vi "Vision Processing.vi"(7 "CameraDevRef":T1) -> ()   [LabVIEW 2011]
doc: "This VI runs in parallel to other tasks. It gets images from the camera, processes them for color or shape and use that information to affect robot behavior."
uses:
  <vilib>/Rock Robotics/WPI/Camera/WPI_CameraDevRef.ctl
  Robot Global Data.vi
  <vilib>/vision/NI_Vision_Development_Module.lvlib
panel:
  out "Distance Array":dbl[](array[numeric])
  out "Distance to Midpoint":dbl
  in  "Scaler":dbl=0.5
  in  "Enable Imaging on Screen":bool
  out "Midpoint":dbl
  in  "Lower Speed Limit":dbl=0.05
  out "Turret Rotation":dbl
  in  "Upper Speed Limit":dbl=0.3
  out "Number of Rectangles Visible":dbl
  out "Y Position Array":dbl[](array[numeric])
  out "X Position Array":dbl[](array[numeric])
  out "Array":T2(array[cluster])
  in  "Score Limits":T3={"Rect Coverage"=76.0, "Aspect Ratio"=40.0, "X Edge Strength"=40.0, "Y Edge Strength"=60.0}
  out "Processed Image":T4(plugin-control)
  out "Original Image":T4(plugin-control)
  in  "Annotate":bool=TRUE
  in  "Particle Count Limit":i32=10
  in  "Area Size Limit":i32=444
  in  "Range":cluster{"Lower value":sgl, "Upper value":sgl}={"Lower value"=120.0, "Upper value"=255.0}
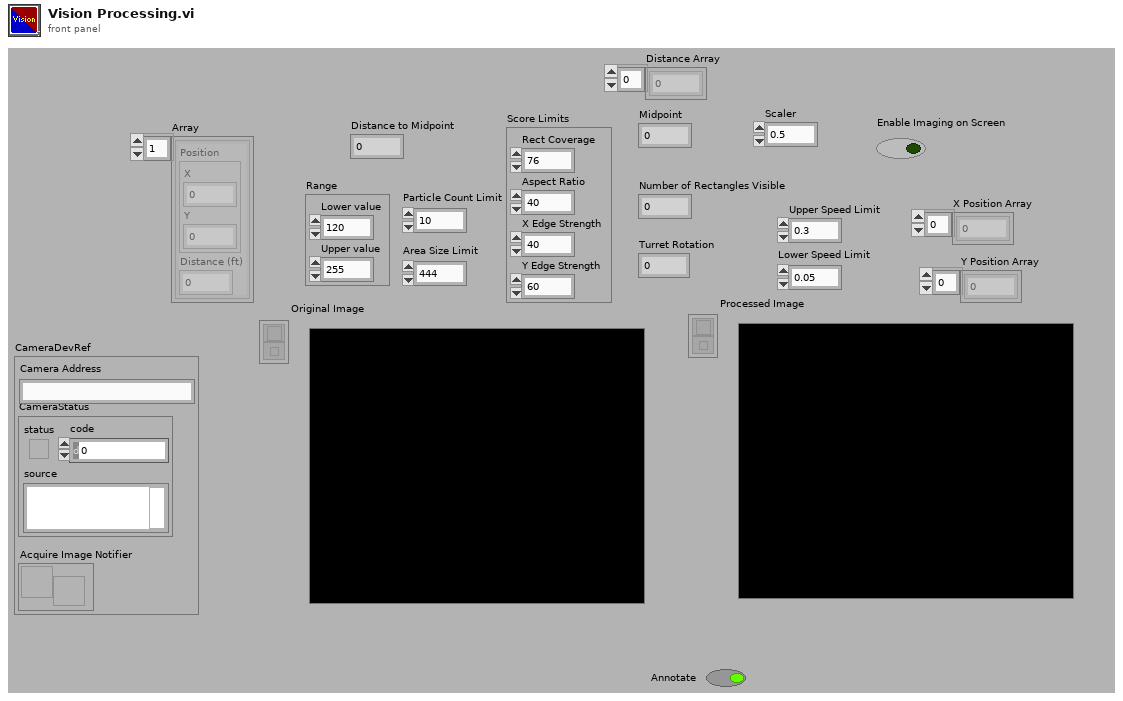
[diagram p1: front panel]
types:
  T1 = typedef "WPI_CameraDevRef.ctl" = cluster{"Camera Address":string, "CameraStatus":errorcluster, "Acquire Image Notifier":refnum<notifier>}
  T2 = cluster{"Position":cluster{"X":dbl, "Y":dbl}, "Distance (ft)":dbl}[]
  T3 = cluster{"Rect Coverage":dbl, "Aspect Ratio":dbl, "X Edge Strength":dbl, "Y Edge Strength":dbl}
  T4 = typedef "IMAQ Image.ctl" = refnum<image>
  T5 = typedef "Image Type" = u32
  T6 = cluster{cluster{"Left":dbl, "Top":dbl, "Right":dbl, "Bottom":dbl}, dbl[]}[]
  T7 = cluster{"Left":dbl, "Top":dbl, "Right":dbl, "Bottom":dbl}
  T8 = cluster{"Target Center (-1 to 1)":cluster{"X":dbl, "Y":dbl}, "Distance (ft)":dbl}
  T9 = cluster{"Target Center (-1 to 1)":cluster{"X":dbl, "Y":dbl}, "Distance (ft)":dbl}[]
  T10 = cluster{"Axis 1":dbl, "Axis 2":dbl, "Axis 3":dbl, "Axis 4":dbl, "Axis 5":dbl, "Axis 6":dbl, "Button 1":bool, "Button 2":bool, "Button 3":bool, "Button 4":bool, "Button 5":bool, "Button 6":bool, "Button 7":bool, "Button 8":bool, "Button 9":bool, "Button 10":bool, "Button 11":bool, "Button 12":bool}
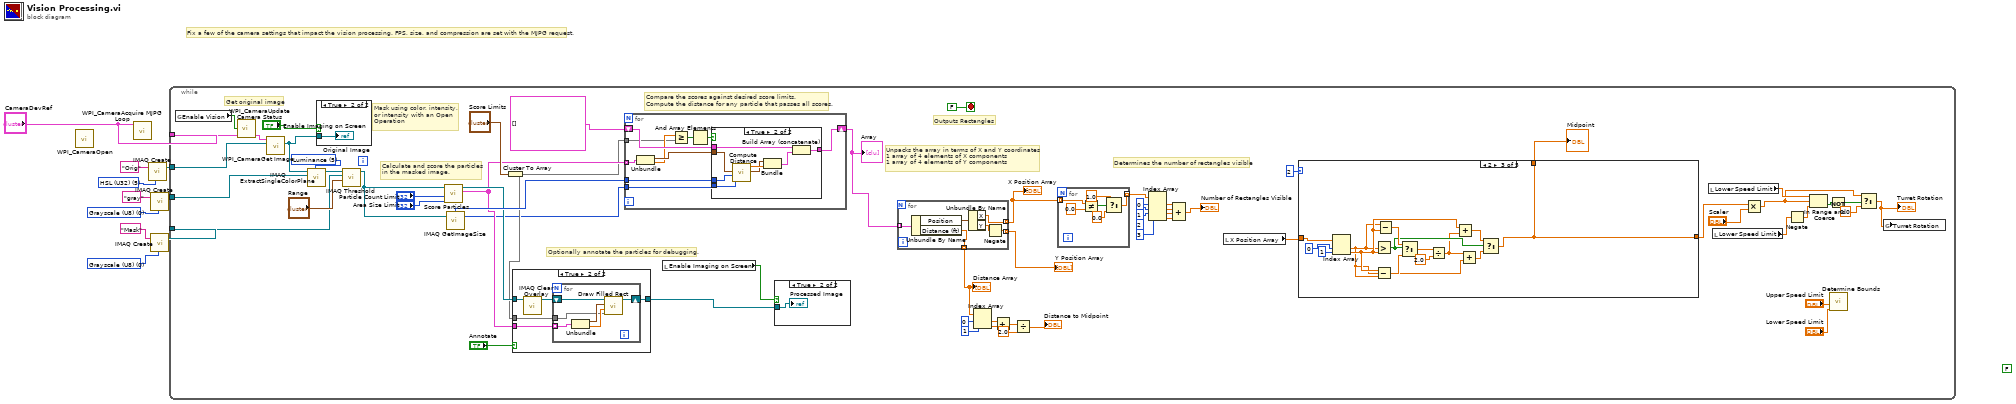
[diagram p0: block diagram]
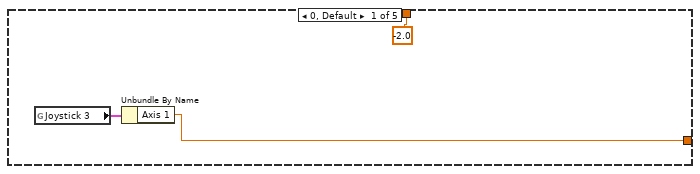
[diagram p4: hidden frame]
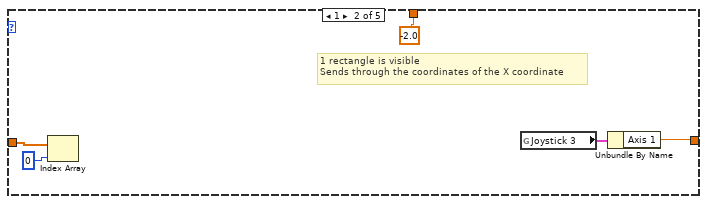
[diagram p5: hidden frame]
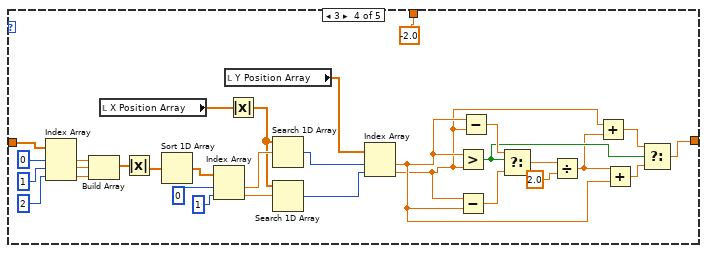
[diagram p6: hidden frame]
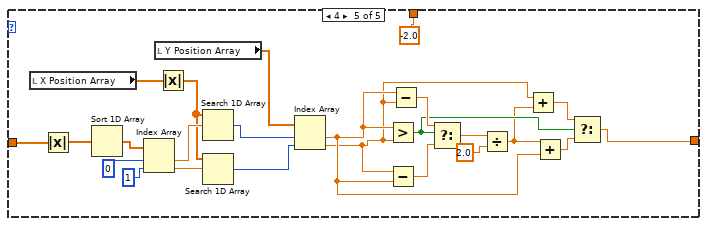
[diagram p7: hidden frame]
diagram:
  w3 = T5 5 items=["Grayscale (U8)", "Grayscale (I16)", "Grayscale (SGL)", "Complex (CSG)", "RGB (U32)", "HSL (U32)", "RGB (U64)", "Grayscale (U16)"] ("Image Type")
  (unwired) FALSE
  w6 = T5 0 items=["Grayscale (U8)", "Grayscale (I16)", "Grayscale (SGL)", "Complex (CSG)", "RGB (U32)", "HSL (U32)", "RGB (U64)", "Grayscale (U16)"] ("Image Type")
  w10 = T5 0 items=["Grayscale (U8)", "Grayscale (I16)", "Grayscale (SGL)", "Complex (CSG)", "RGB (U32)", "HSL (U32)", "RGB (U64)", "Grayscale (U16)"] ("Image Type")
  # "Fix a few of the camera settings that impact the vision processing. FPS, size, and compression are set with the MJPG request."
  n1 = call <vilib>:"WPI_CameraOpen.vi"() -> ()  [unwired: 10 in, 2 out]
  n2 = call <vilib>:"WPI_CameraAcquire MJPG Loop.vi"("CameraDevRef"="CameraDevRef") -> ()  [unwired: 11 in]
  n3 = call "IMAQ Create"("Image Name"="Orig", "Image Type"=w3) -> ("New Image"=w2:T4)  [unwired: 2 in, 2 out]
  n4 = call "IMAQ Create"("Image Name"="gray", "Image Type"=w10) -> ("New Image"=w8:T4)  [unwired: 2 in, 2 out]
  n5 = call "IMAQ Create"("Image Name"="Mask", "Image Type"=w6) -> ("New Image"=w5:T4)  [unwired: 2 in, 2 out]
  n6 = while {
    tunnel: w8 -> [w56]
    tunnel: w5 -> [w57]
    tunnel: w2 -> [w35]
    tunnel: "CameraDevRef" -> [w33]
    stop <- FALSE stop-if-true
    w60 = 5 items=["Red", "Green", "Blue", "Hue", "Saturation", "Luminance", "Value", "Intensity"] ("Color Plane")
    # "Determines the number of rectangles visible"
    # "Unpacks the array in terms of X and Y coordinates\n1 array of 4 elements of X components\n1 array of 4 elements of Y components"
    # "Outputs Rectangles"
    # "Optionally annotate the particles for debugging."
    # "Compare the scores against desired score limits.\nCompute the distance for any particle that passes all scores."
    # "Calculate and score the particles\nin the masked image."
    # "Mask using color, intensity,\nor intensity with an Open\nOperation"
    # "Get original image"
    n7 = global read "Robot Global Data.vi" "Enable Vision"() -> (w32:bool)
    n8 = call <vilib>:"WPI_CameraUpdate Camera Status.vi"("CameraDevRef In"=w33, "Enable Vision"=w32) -> ("CameraDevRef Out"=w34:T1)  [unwired: 3 in]
    n9 = call <vilib>:"WPI_CameraGet Image.vi"("Image"=w35, "CameraDevRef"=w34) -> ("Image Out"=w31:T4)  [unwired: 7 in, 2 out]
    n10 = call "IMAQ ExtractSingleColorPlane"("Color Plane"=w60, "Image Dst"=w56, "Image Src"=w31) -> ("Image Dst Out"=w58:T4)  [unwired: 1 in, 7 out]
    n11 = case shown="True" "Enable Imaging on Screen" {
      tunnel: w31 -> [_ w73]
      frame False {
      }
      frame True {
        "Original Image" <- w73
      }
    }
    n12 = call "IMAQ Threshold"("Range"="Range", "Image Dst"=w57, "Image Src"=w58) -> ("Image Dst Out"=w55:T4)  [unwired: 3 in, 5 out]
    n13 = call "Score Particles.vi"("Area Size Limit"="Area Size Limit", "Particle Count Limit"="Particle Count Limit", "Image Refnum in"=w55) -> ("Scored Particle Info"=w67:T6, "Image Refnum out"=w70:T4)  [unwired: 7 in]
    n14 = call "IMAQ GetImageSize"("Image"=w55) -> ("Y Resolution"=w61:i32, "X Resolution"=w71:i32)  [unwired: 3 in, 1 out]
    n15 = Cluster To Array(cluster="Score Limits") -> (array=w65:dbl[])
    n16 = case shown="True" "Annotate" {
      tunnel: w70 -> [w163 w168]
      tunnel: [w163 w167] -> w68
      tunnel: w67 -> [_ w165]
      tunnel: w65 -> [_ w164]
      frame False {
      }
      frame True {
        n17 = call "IMAQ Clear Overlay"("Image"=w168) -> ("Image Out"=w166:T4)  [unwired: 2 in, 8 out]
        n18 = for {
          shift-right: [w173] -> w167
          shift-left: w166 -> [w174]
          tunnel: w165 -> [w170] mode=indexing
          tunnel: w164 -> [w169]
          n19 = Unbundle(w170) -> (w171:T7, w172:dbl[])
          n20 = call "Draw Filled Rect.vi"("Limits"=w169, "Scores"=w172, "Bounding Box"=w171, "image in"=w174) -> ("image out"=w173:T4)  [unwired: 7 in]
        }
      }
    }
    n21 = for {
      shift-right: [w183] -> w36
      shift-left: T2 [] -> [w184]
      tunnel: w71 -> [w182]
      tunnel: w67 -> [w180] mode=indexing
      tunnel: w65 -> [w176]
      tunnel: w61 -> [w175]
      n22 = Unbundle(w180) -> (w181:T7, w177:dbl[])
      n23 = Greater Or Equal?(x=w177, y=w176) -> (x >= y?=w179:bool[])
      n24 = And Array Elements(Boolean array=w179) -> (logical AND=w178:bool)
      n25 = case shown="True" w178 {
        tunnel: w184 -> [w185 w193]
        tunnel: [w185 w192] -> w183
        tunnel: w181 -> [_ w188]
        tunnel: w182 -> [_ w190]
        tunnel: w175 -> [_ w186]
        frame False {
        }
        frame True {
          n26 = call "Compute Distance.vi"("Y Image Resolution"=w186, "X Image Resolution"=w190, "Bounding Box"=w188) -> ("Target Center (-1 to 1)"=w187:cluster{"X":dbl, "Y":dbl}, "Distance (ft)"=w189:dbl)  [unwired: 7 in]
          n27 = Bundle("Target Center (-1 to 1)"=w187, "Distance (ft)"=w189) -> (w191:T8)  [unwired: 1 in]
          n28 = Build Array (concatenate)(w193, w191) -> (w192:T9)
        }
      }
    }
    "Array" <- w36
    n29 = local read "Enable Imaging on Screen"() -> (w29:bool)
    n30 = case shown="True" w29 {
      tunnel: w68 -> [_ w72]
      frame False {
      }
      frame True {
        "Processed Image" <- w72
      }
    }
    n31 = for {
      tunnel: [w160] -> w49 mode=indexing
      tunnel: [w161] -> w38 mode=indexing
      tunnel: w36 -> [w158] mode=indexing
      tunnel: [w157] -> w18 mode=indexing
      n32 = Unbundle By Name(w158) -> ("Position"=w162:cluster{"X":dbl, "Y":dbl}, "Distance (ft)"=w157:dbl)
      n33 = Unbundle By Name(w162) -> ("X"=w161:dbl, "Y"=w159:dbl)
      n34 = Negate(x=w159) -> (-x=w160:dbl)
    }
    "X Position Array" <- w38
    "Y Position Array" <- w49
    "Distance Array" <- w18
    n35 = Index Array(array=w18, index #1=0 ("index"), index #2=1 ("index")) -> (element #1=w14:dbl, element #2=w15:dbl)
    n36 = Add(x=w14, y=w15) -> (x+y=w13:dbl)
    n37 = Divide(x=w13, y=2.0) -> (x/y=→"Distance to Midpoint":dbl)
    n38 = for {
      tunnel: w38 -> [w78] mode=indexing
      tunnel: [w74] -> w39 mode=indexing
      n39 = Not Equal?(x=w78, y=0.0) -> (x != y?=w77:bool)
      n40 = Select(t=1.0, s=w77, f=0.0) -> (s? t:f=w74:dbl)
    }
    n41 = Index Array(array=w39, index #1=0 ("index"), index #2=1 ("index"), index #3=2 ("index"), index #4=3 ("index")) -> (element #1=w41:dbl, element #2=w40:dbl, element #3=w42:dbl, element #4=w43:dbl)
    n42 = Compound Arithmetic op=ADD(w41, w40, w42, w43) -> (→"Number of Rectangles Visible":dbl)
    n43 = local read "X Position Array"() -> (w37:dbl[])
    n44 = case shown="2" 2 {
      tunnel: w37 -> [_ w87 w101 w132 w136]
      tunnel: [w81 w84 w88 w104 w135] -> w22
      tunnel: [-2.0 -2.0 w88 -2.0 -2.0] -> w52
      frame 0, Default {
        n45 = global read "Robot Global Data.vi" "Joystick 3"() -> (w82:T10)
        n46 = Unbundle By Name(w82) -> ("Axis 1"=w81:dbl)
      }
      frame 1 {
        # "1 rectangle is visible\nSends through the coordinates of the X coordinate"
        n47 = Index Array(array=w87, index=0) -> ()  [unwired: 1 out]
        n48 = global read "Robot Global Data.vi" "Joystick 3"() -> (w85:T10)
        n49 = Unbundle By Name(w85) -> ("Axis 1"=w84:dbl)
      }
      frame 2 {
        n50 = Index Array(array=w101, index #1=0 ("index"), index #2=1 ("index")) -> (element #1=w89:dbl, element #2=w90:dbl)
        n51 = Greater?(x=w89, y=w90) -> (0:w94:bool)
        n52 = Subtract(x=w90, y=w89) -> (x-y=w97:dbl)
        n53 = Subtract(x=w89, y=w90) -> (x-y=w98:dbl)
        n54 = Select(t=w98, s=w94, f=w97) -> (s? t:f=w96:dbl)
        n55 = Divide(x=w96, y=2.0) -> (x/y=w91:dbl)
        n56 = Add(x=w90, y=w91) -> (x+y=w93:dbl)
        n57 = Add(x=w91, y=w89) -> (x+y=w92:dbl)
        n58 = Select(t=w93, s=w94, f=w92) -> (s? t:f=w88:dbl)
      }
      frame 3 {
        n59 = Index Array(array=w132, index #1=0 ("index"), index #2=1 ("index"), index #3=2 ("index")) -> (element #1=w128:dbl, element #2=w127:dbl, element #3=w126:dbl)
        n60 = Build Array(w128, w127, w126) -> (w125:dbl[])
        n61 = local read "X Position Array"() -> (w118:dbl[])
        n62 = Absolute Value(x=w125) -> (abs(x)=w124:dbl[])
        n63 = Sort 1D Array(array=w124) -> (sorted array=w123:dbl[])
        n64 = Index Array(array=w123, index #1=0 ("index"), index #2=1 ("index")) -> (element #1=w120:dbl, element #2=w119:dbl)
        n65 = local read "Y Position Array"() -> (w116:dbl[])
        n66 = Absolute Value(x=w118) -> (abs(x)=w103:dbl[])
        n67 = Search 1D Array(1D array=w103, element=w120) -> (index of element=w117:i32)  [unwired: 1 in]
        n68 = Search 1D Array(1D array=w103, element=w119) -> (index of element=w115:i32)  [unwired: 1 in]
        n69 = Index Array(array=w116, index #1=w117, index #2=w115) -> (element #1=w106:dbl, element #2=w105:dbl)
        n70 = Greater?(x=w106, y=w105) -> (0:w110:bool)
        n71 = Subtract(x=w105, y=w106) -> (x-y=w113:dbl)
        n72 = Subtract(x=w106, y=w105) -> (x-y=w114:dbl)
        n73 = Select(t=w114, s=w110, f=w113) -> (s? t:f=w112:dbl)
        n74 = Divide(x=w112, y=2.0) -> (x/y=w107:dbl)
        n75 = Add(x=w105, y=w107) -> (x+y=w109:dbl)
        n76 = Add(x=w107, y=w106) -> (x+y=w108:dbl)
        n77 = Select(t=w109, s=w110, f=w108) -> (s? t:f=w104:dbl)
      }
      frame 4 {
        n78 = local read "X Position Array"() -> (w150:dbl[])
        n79 = Absolute Value(x=w136) -> (abs(x)=w156:dbl[])
        n80 = Sort 1D Array(array=w156) -> (sorted array=w155:dbl[])
        n81 = Index Array(array=w155, index #1=0 ("index"), index #2=1 ("index")) -> (element #1=w152:dbl, element #2=w151:dbl)
        n82 = local read "Y Position Array"() -> (w148:dbl[])
        n83 = Absolute Value(x=w150) -> (abs(x)=w134:dbl[])
        n84 = Search 1D Array(1D array=w134, element=w152) -> (index of element=w149:i32)  [unwired: 1 in]
        n85 = Search 1D Array(1D array=w134, element=w151) -> (index of element=w147:i32)  [unwired: 1 in]
        n86 = Index Array(array=w148, index #1=w149, index #2=w147) -> (element #1=w138:dbl, element #2=w137:dbl)
        n87 = Greater?(x=w138, y=w137) -> (0:w142:bool)
        n88 = Subtract(x=w137, y=w138) -> (x-y=w145:dbl)
        n89 = Subtract(x=w138, y=w137) -> (x-y=w146:dbl)
        n90 = Select(t=w146, s=w142, f=w145) -> (s? t:f=w144:dbl)
        n91 = Divide(x=w144, y=2.0) -> (x/y=w139:dbl)
        n92 = Add(x=w137, y=w139) -> (x+y=w141:dbl)
        n93 = Add(x=w139, y=w138) -> (x+y=w140:dbl)
        n94 = Select(t=w141, s=w142, f=w140) -> (s? t:f=w135:dbl)
      }
    }
    "Midpoint" <- w52
    n95 = local read "Lower Speed Limit"() -> (w25:dbl)
    n96 = local read "Lower Speed Limit"() -> (w27:dbl)
    n97 = Multiply(x=w22, y="Scaler") -> (x*y=w19:dbl)
    n98 = Negate(x=w27) -> (-x=w26:dbl)
    n99 = In Range and Coerce(upper limit=w25, x=w19, lower limit=w26) -> (In Range?=w24:bool)  [unwired: 1 out]
    n100 = Not(x=w24) -> (.not. x?=w23:bool)
    n101 = call "Determine Bounds.vi"("Lower Limit"="Lower Speed Limit", "Upper Limit"="Upper Speed Limit") -> ()  [unwired: 9 in, 1 out]
    n102 = Select(t=w19, s=w23, f=0.0) -> (s? t:f=w20:dbl)
    "Turret Rotation" <- w20
    n103 = global write "Robot Global Data.vi" "Turret Rotation"(w20) -> ()
  }
